vi "Data_Analysis_GUI.vi"() -> ()   [LabVIEW 2019]
uses:
  <vilib>/Utility/error.llb/DialogType.ctl
  Data Analysis/Data_Analysis_Global_var.vi
  <vilib>/Utility/Data Type/NI_Data Type.lvlib
panel:
  in  "Delay (ns)":dbl
  in  "Attenuation":dbl
  out "Scope 2":waveform(dbl)[](graph)
  out "Scope":waveform(dbl)[](graph)
  in  "Filter Data":bool
  out "Processing":bool
  out "FileList":string[](array[string])
  in  "Update":bool
  in  "File Contents":string[](tree)
  in  "Clear List":bool
  out "Loaded Files":string[](array[string])
  out "Min Value":i32
  in  "Stop":bool
  in  "Add File":bool
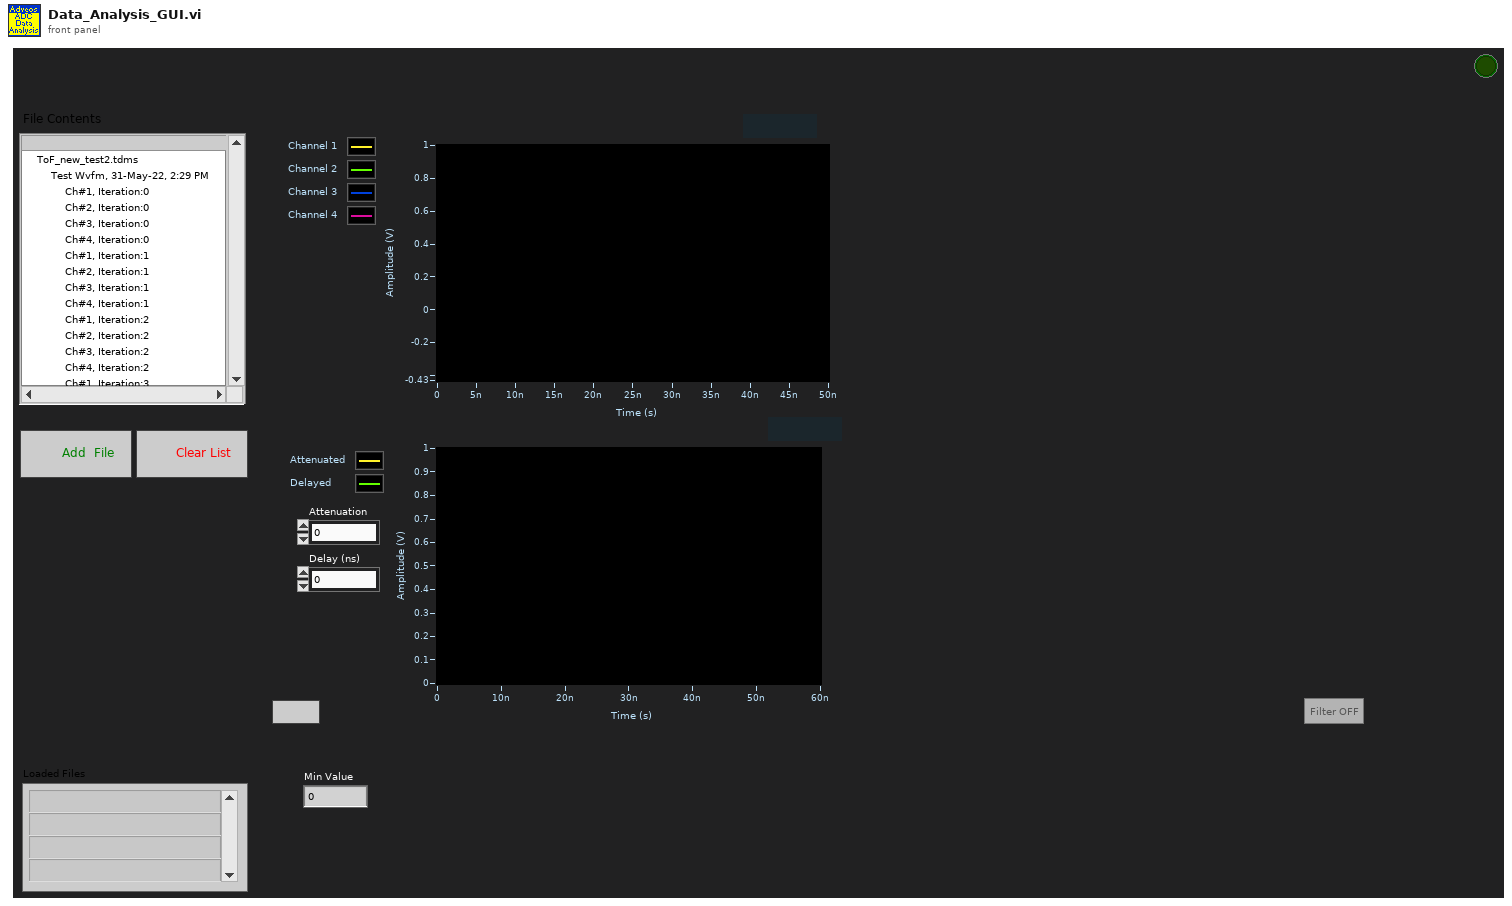
[diagram p1: front panel]
types:
  T1 = enum16{"open", "open or create", "create or replace", "create", "open (read-only)"}
  T2 = typedef "DialogType.ctl" = u16
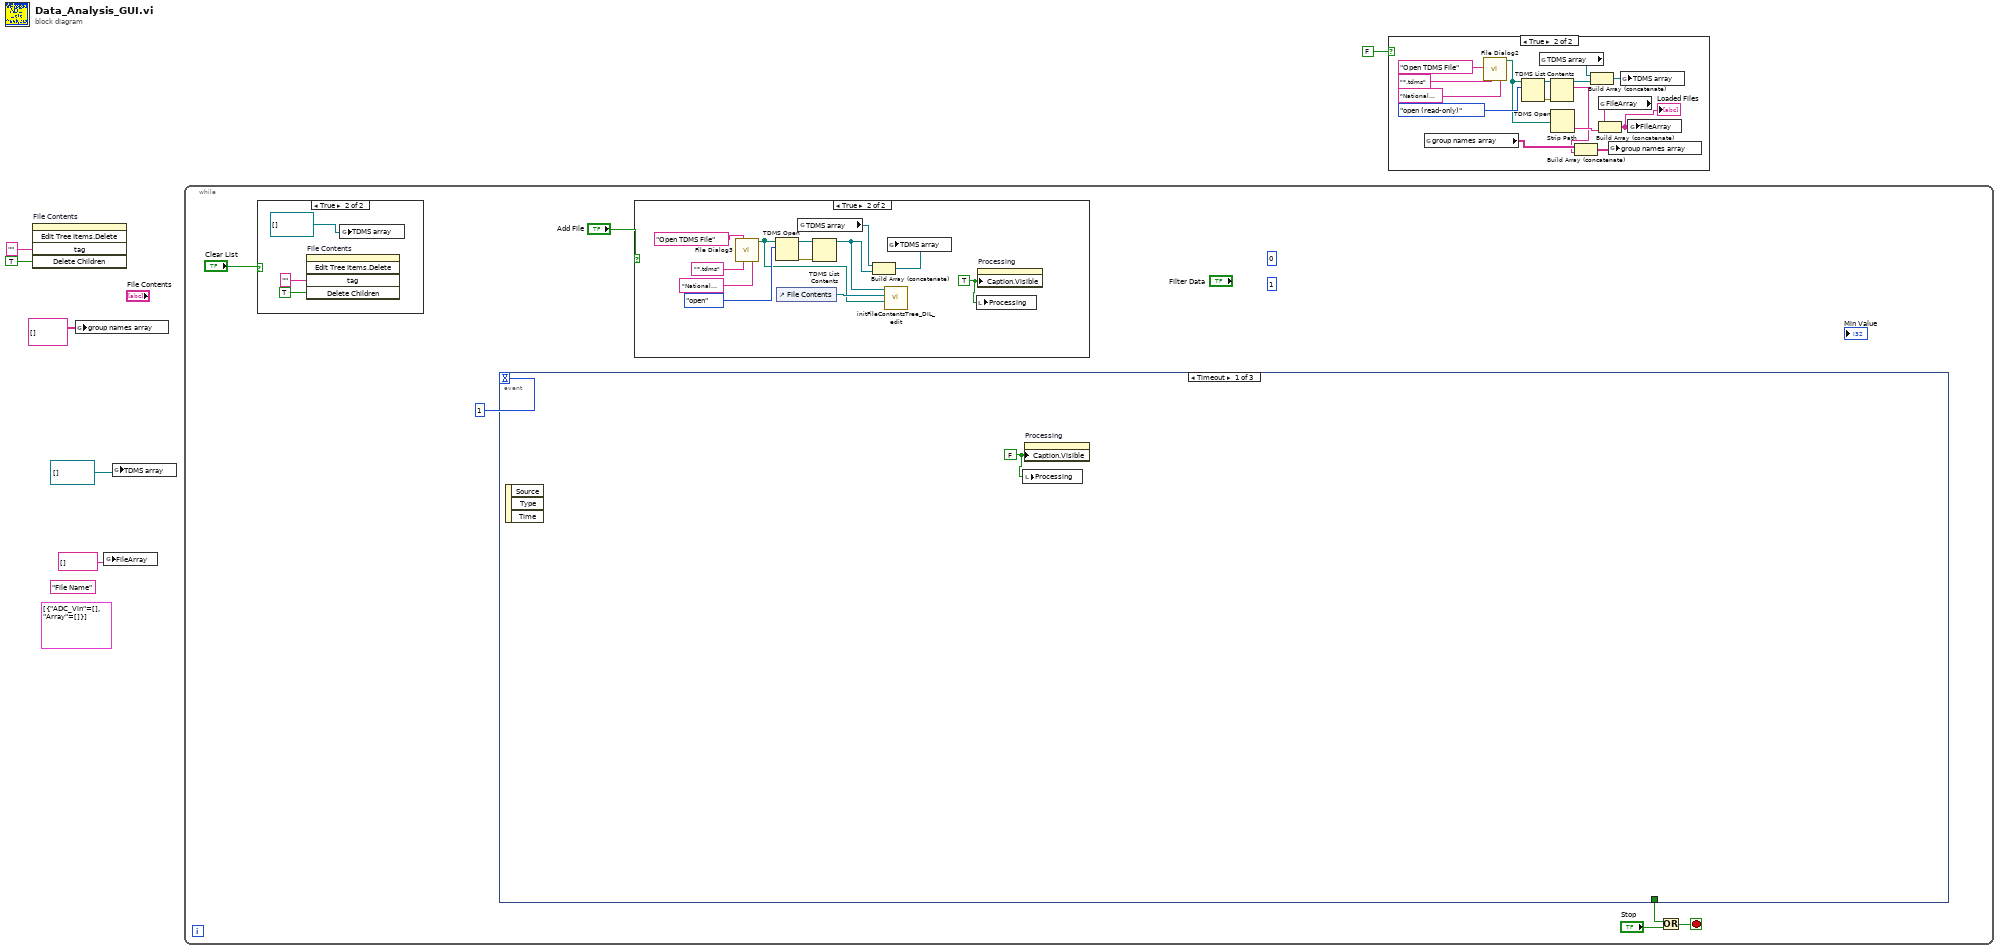
[diagram p0: block diagram]
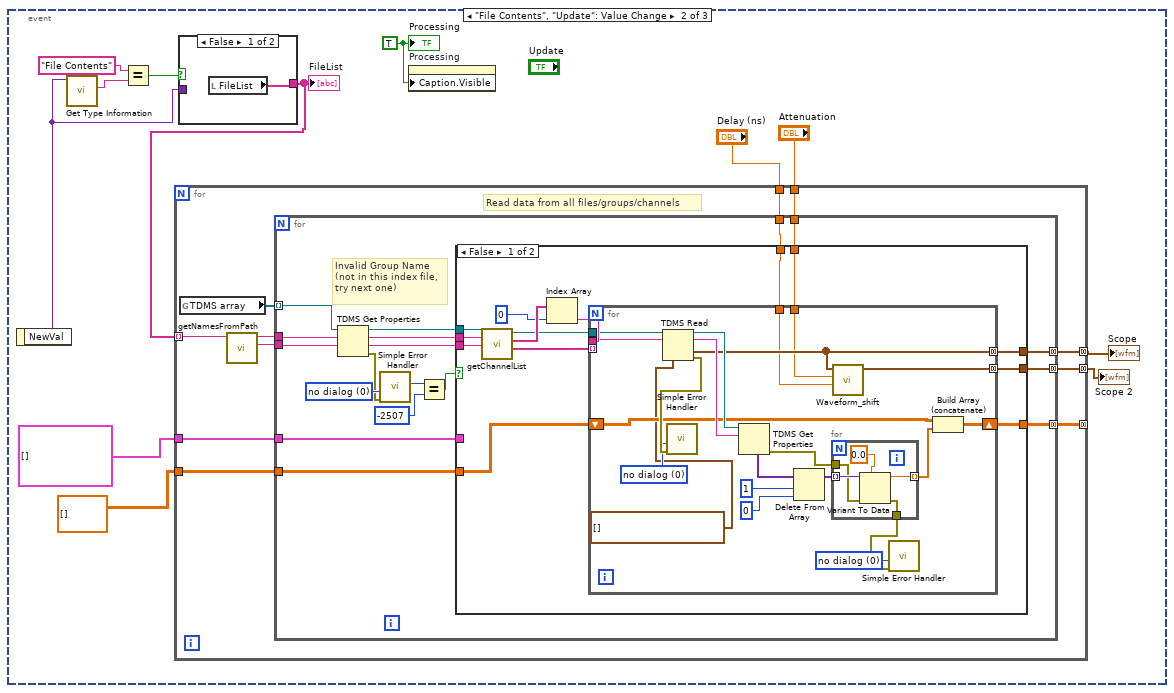
[diagram p5: hidden frame]
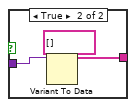
[diagram p6: hidden frame]
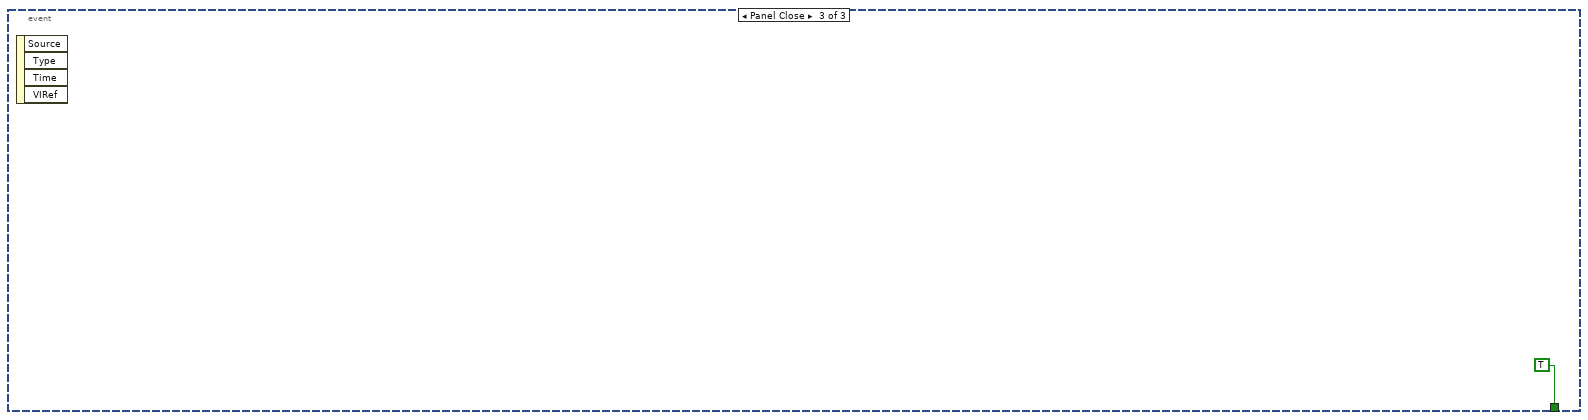
[diagram p8: hidden frame]
diagram:
  (unwired) cluster{"ADC_Vin":u32[], "Array":u16[]}[] [{"ADC_Vin"=[], "Array"=[]}] ("XY Graph")
  (unwired) "File Name" ("Caption.Text")
  n1 = invoke on="File Contents" class="Tree (strict)" method="Edit Tree Items.Delete"("tag"="" ("Tag"), "Delete Children"=TRUE ("Delete Children?")) -> ()  [unwired: 3 in, 5 out]
  n2 = global write "Data_Analysis_Global_var.vi" "group names array"(string[][] [] ("group names array")) -> ()
  n3 = global write "Data_Analysis_Global_var.vi" "FileArray"(string[] [] ("Item Names")) -> ()
  n4 = global write "Data_Analysis_Global_var.vi" "TDMS array"(refnum<k34>[] [] ("TDMS array")) -> ()
  n5 = while {
    stop <- w11 stop-if-true
    (unwired) u32 1 ("Active Cursor")
    (unwired) u32 0 ("Active Cursor")
    n6 = case shown="True" "Clear List" {
      frame False {
      }
      frame True {
        n7 = invoke on="File Contents" class="Tree (strict)" method="Edit Tree Items.Delete"("tag"="" ("Tag"), "Delete Children"=TRUE ("Delete Children?")) -> ()  [unwired: 3 in, 5 out]
        n8 = global write "Data_Analysis_Global_var.vi" "TDMS array"(refnum<k34>[] [] ("Tdms file array")) -> ()
      }
    }
    n9 = event shown="[0] Timeout" {
      selector: _ -> [_ _ _]
      dyn-events: _ -> [_ _ _]
      timeout: 1 -> [_ _ _]
      tunnel: [_ _ TRUE] -> w10
      event Timeout {
        w28 = FALSE ("Caption.Visible")
        n10 = event-data() -> ()  [unwired: 1 in, 3 out]
        n11 = local write "Processing"(w28) -> ()
        n12 = property on="Processing" class="Bool (strict)"("Caption.Visible"=w28) -> ()  [unwired: 2 in, 2 out]
      }
      event "File Contents", "Update": Value Change {
        w33 = TRUE ("Processing")
        n13 = event-data() -> ("NewVal"=w35:variant)  [unwired: 1 in]
        n14 = call <vilib>:"Get Type Information.vi"("variant"=w35) -> ("name"=w38:string)  [unwired: 6 in, 4 out]
        n15 = Equal?(x="File Contents", y=w38) -> (x = y?=w36:bool)
        n16 = case shown="False" w36 {
          tunnel: w35 -> [_ w43]
          tunnel: [w41 w42] -> w34
          frame False {
            n17 = local read "FileList"() -> (w41:string[])
          }
          frame True {
            n18 = Variant To Data(type=string[] [], Variant=w43) -> (data=w42:string[])  [unwired: 1 in, 1 out]
          }
        }
        "FileList" <- w34
        n19 = for {
          tunnel: w34 -> [w55] mode=indexing
          tunnel: [w51] -> _ mode=concatenating
          tunnel: cluster{u16[], u16[]}[] [] -> [w50]
          tunnel: dbl[][] [] -> [w49]
          tunnel: [w48] -> w32 mode=concatenating
          tunnel: [w47] -> w31 mode=concatenating
          tunnel: "Attenuation" -> [w46]
          tunnel: "Delay (ns)" -> [w45]
          # "Read data from all files/groups/channels"
          n20 = global read "Data_Analysis_Global_var.vi" "TDMS array"() -> (w52:refnum<k34>[])
          n21 = call <vilib>:"getNamesFromPath.vi"("tree path"=w55) -> ("channel"=w53:string, "group"=w54:string)  [unwired: 1 in, 4 out]
          n22 = for {
            tunnel: w54 -> [w69]
            tunnel: w53 -> [w68]
            tunnel: w52 -> [w66] mode=indexing
            tunnel: [w62] -> w51 mode=concatenating
            tunnel: w50 -> [w61]
            tunnel: w49 -> [w60]
            tunnel: [w59] -> w48 mode=concatenating
            tunnel: [w58] -> w47 mode=concatenating
            tunnel: w46 -> [w57]
            tunnel: w45 -> [w56]
            w73 = T2 0 items=["no dialog", "OK message", "continue or stop message", "OK message + warnings", "continue/stop + warnings"] ("type of dialog (OK msg:1)")
            # "Invalid Group Name\n(not in this index file,\ntry next one)"
            n23 = TDMS Get Properties(9:w68, 10:w69, 11:w66) -> (0:w72:errorcluster, 1:w63:string, 2:w64:string, 3:w65:refnum<k34>)  [unwired: 1 in, 4 out]
            n24 = call <vilib>:"Simple Error Handler.vi"("type of dialog (OK msg:1)"=w73, "error in (no error)"=w72) -> ("code out"=w71:i32)  [unwired: 3 in, 4 out]
            n25 = Equal?(x=w71, y=-2507) -> (x = y?=w67:bool)
            n26 = case shown="False" w67 {
              tunnel: w65 -> [w85 _]
              tunnel: w64 -> [w84 _]
              tunnel: w63 -> [w83 _]
              tunnel: [w79 w114] -> w62
              tunnel: w61 -> [_ _]
              tunnel: w60 -> [w78 w114]
              tunnel: [w77 _] -> w59
              tunnel: [w76 _] -> w58
              tunnel: w57 -> [w75 _]
              tunnel: w56 -> [w74 _]
              frame False {
                n27 = call <vilib>:"getChannelList.vi"("channel names"=w83, "group name"=w84, "tdms file"=w85) -> ("channel names out"=w80:string[], "group names out"=w87:string[], "tdms file out"=w81:refnum<k34>)  [unwired: 1 in, 1 out]
                n28 = Index Array(array=w87, index=0) -> (element=w82:string)
                n29 = for {
                  tunnel: w82 -> [w107]
                  tunnel: w81 -> [w108]
                  tunnel: w80 -> [_] mode=indexing
                  shift-right: [w94] -> w79
                  shift-left: w78 -> [w93]
                  tunnel: [w91] -> w77 mode=concatenating
                  tunnel: [w90] -> w76 mode=concatenating
                  tunnel: w75 -> [w89]
                  tunnel: w74 -> [w88]
                  w96 = T2 0 items=["no dialog", "OK message", "continue or stop message", "OK message + warnings", "continue/stop + warnings"] ("type of dialog (OK msg:1)")
                  w102 = T2 0 items=["no dialog", "OK message", "continue or stop message", "OK message + warnings", "continue/stop + warnings"] ("type of dialog (OK msg:1)")
                  n30 = TDMS Read(0:w108, 5:w107, 12:waveform(dbl)[] [] ("appended array")) -> (4:w99:refnum<k34>, 6:w98:string, 10:w91:waveform(dbl)[], 15:w97:errorcluster)  [unwired: 5 in, 2 out]
                  n31 = call <vilib>:"Simple Error Handler.vi"("type of dialog (OK msg:1)"=w96, "error in (no error)"=w97) -> ()  [unwired: 3 in, 5 out]
                  n32 = TDMS Get Properties(10:w98, 11:w99) -> (0:w105:errorcluster, 4:w104:variant[])  [unwired: 2 in, 6 out]
                  n33 = Delete From Array(array=w104, length=1, index=0 ("length")) -> (array with subset deleted=w103:variant[])  [unwired: 1 out]
                  n34 = for {
                    tunnel: [w113] -> w95 mode=indexing
                    tunnel: w103 -> [w112] mode=indexing
                    tunnel: [w110] -> w106
                    tunnel: w105 -> [w109]
                    n35 = Variant To Data(error in=w109, type=0.0, Variant=w112) -> (data=w113:dbl, error out=w110:errorcluster)
                  }
                  n36 = call "Waveform_shift.vi"("Delay (ns)"=w88, "Attenuation"=w89, "Waveform_in"=w91) -> ("Wavefrom_out"=w90:waveform(dbl)[])  [unwired: 8 in]
                  n37 = call <vilib>:"Simple Error Handler.vi"("type of dialog (OK msg:1)"=w102, "error in (no error)"=w106) -> ()  [unwired: 3 in, 5 out]
                  n38 = Build Array (concatenate)(w93, w95) -> (w94:dbl[][])
                }
              }
              frame True {
              }
            }
          }
        }
        "Scope" <- w32
        "Scope 2" <- w31
        n39 = property on="Processing" class="Bool (strict)"("Caption.Visible"=w33) -> ()  [unwired: 2 in, 2 out]
        "Processing" <- w33
      }
      event Panel Close {
        n40 = event-data() -> ()  [unwired: 1 in, 4 out]
      }
    }
    n41 = case shown="True" "Add File" {
      frame False {
      }
      frame True {
        w13 = TRUE ("Caption.Visible")
        n42 = call "File Dialog3"("prompt"="Open TDMS File" ("prompt tdms"), "pattern (all files)"="*.tdms", "pattern label"="National Instruments TDM Streaming" ("pattern label tdms")) -> ("selected path"=w17:path)  [unwired: 4 in, 8 out]
        n43 = TDMS Open(10:T1."open" ("operation (0:open)"), 11:w17) -> (0:w19:errorcluster, 3:w20:refnum<k34>)  [unwired: 5 in]
        n44 = control-ref of="File Contents"() -> (w18:refnum<vi>)
        n45 = global read "Data_Analysis_Global_var.vi" "TDMS array"() -> (w15:refnum<k34>[])
        n46 = TDMS List Contents(4:w19, 7:w20) -> (3:w16:refnum<k34>)  [unwired: 1 in, 3 out]
        n47 = Build Array (concatenate)(w15, w16) -> (w14:refnum<k34>[])
        n48 = call "initFileContentsTree_DIL_edit.vi"("file path"=w17, "Tree Refnum"=w18, "tdms file"=w16) -> ()  [unwired: 3 in, 2 out]
        n49 = global write "Data_Analysis_Global_var.vi" "TDMS array"(w14) -> ()
        n50 = local write "Processing"(w13) -> ()
        n51 = property on="Processing" class="Bool (strict)"("Caption.Visible"=w13) -> ()  [unwired: 2 in, 2 out]
      }
    }
    n52 = Or(x=w10, y="Stop") -> (x .or. y?=w11:bool)
  }
  n53 = case shown="True" FALSE {
    frame False {
    }
    frame True {
      n54 = global read "Data_Analysis_Global_var.vi" "group names array"() -> (w118:string[][])
      n55 = call "File Dialog2"("prompt"="Open TDMS File" ("prompt tdms"), "pattern (all files)"="*.tdms", "pattern label"="National Instruments TDM Streaming" ("pattern label tdms")) -> ("selected path"=w122:path)  [unwired: 4 in, 8 out]
      n56 = TDMS Open(10:T1."open (read-only)" ("operation (0:open)"), 11:w122) -> (0:w127:errorcluster, 3:w126:refnum<k34>)  [unwired: 5 in]
      n57 = global read "Data_Analysis_Global_var.vi" "TDMS array"() -> (w124:refnum<k34>[])
      n58 = TDMS List Contents(4:w127, 7:w126) -> (2:w117:string[], 3:w125:refnum<k34>)  [unwired: 1 in, 2 out]
      n59 = Strip Path(path=w122) -> (name=w120:string)  [unwired: 1 out]
      n60 = Build Array (concatenate)(w118, w117) -> (w116:string[][])
      n61 = Build Array (concatenate)(w124, w125) -> (w123:refnum<k34>[])
      n62 = global read "Data_Analysis_Global_var.vi" "FileArray"() -> (w121:string[])
      n63 = Build Array (concatenate)(w121, w120) -> (w119:string[])
      "Loaded Files" <- w119
      n64 = global write "Data_Analysis_Global_var.vi" "group names array"(w116) -> ()
      n65 = global write "Data_Analysis_Global_var.vi" "TDMS array"(w123) -> ()
      n66 = global write "Data_Analysis_Global_var.vi" "FileArray"(w119) -> ()
    }
  }
